vi "TCP Send MessageHead.vi"(8 "error in (no error)":errorcluster, 9 "Array":i16[](array[numeric]), 11 "connection ID":refnum<k5>) -> (0 "error out":errorcluster)   [LabVIEW 2011]
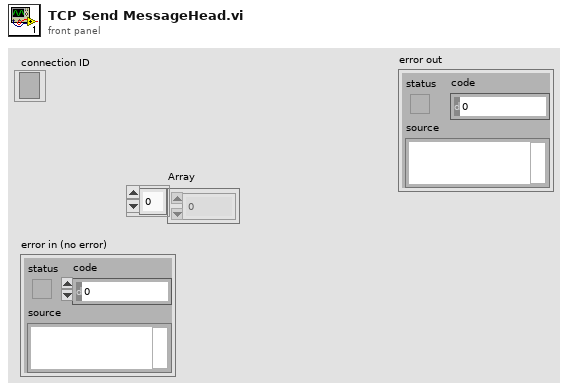
[diagram p1: front panel]
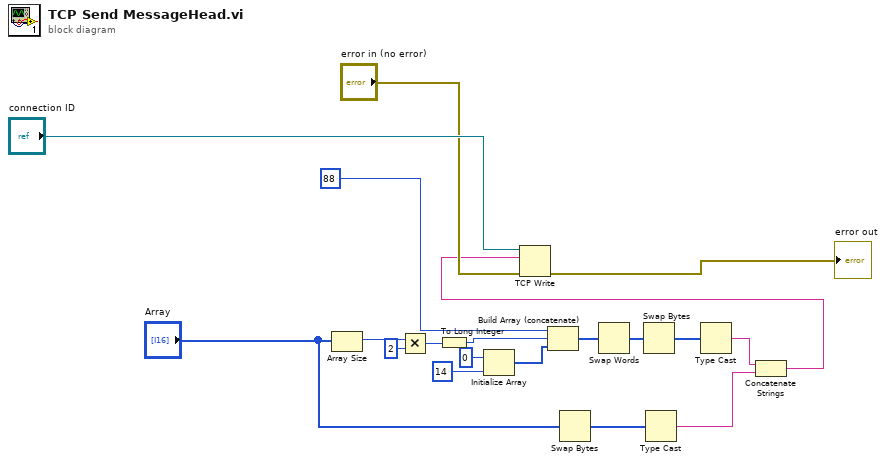
[diagram p0: block diagram]
diagram:
  n1 = Array Size(array="Array") -> (size(s)=w8:i32)
  n2 = Multiply(x=w8, y=2) -> (x*y=w6:i32)
  n3 = To Long Integer(number=w6) -> (32bit integer=w1:i32)
  n4 = Initialize Array(0, 14 ("dimension size")) -> (w13:i32[])
  n5 = Build Array (concatenate)(88, w1, w13) -> (w3:i32[])
  n6 = Swap Bytes(anything="Array") -> (byte swapped=w5:i16[])
  n7 = Swap Words(1:w3) -> (0:w19:i32[])
  n8 = Swap Bytes(anything=w19) -> (byte swapped=w2:i32[])
  n9 = Type Cast(x=w5) -> (*(type *) &x=w11:string)  [unwired: 1 in]
  n10 = Type Cast(x=w2) -> (*(type *) &x=w12:string)  [unwired: 1 in]
  n11 = Concatenate Strings(w12, w11) -> (w10:string)
  n12 = TCP Write(connection ID="connection ID", data in=w10, error in (no error)="error in (no error)") -> (error out=→"error out":errorcluster)  [unwired: 1 in, 2 out]
